vi "Helium Test - Step 2.vi"(7 "Step":i32, 8 "error in":errorcluster, 9 "Test Results":T9, 10 "Oil In":T1, 11 "Test Configuration":T2) -> (0 "error out":errorcluster, 1 "Test Results Out":T9, 2 "Oil Out":T1, 3 "Test Configuration Out":T2)   [LabVIEW 2015]
uses:
  Controls/Test Results.ctl
  Controls/Step Result.ctl
  Controls/Startup Test.ctl
  Controls/Test Information.ctl
  Controls/Vacuum Test.ctl
  Controls/Test Timing.ctl
  Controls/Vaccum Thresholds.ctl
  Controls/Helium Test.ctl
  Controls/Helium Thresholds.ctl
  Controls/Startup Thresholds.ctl
  CAN Communication/Oil/Typedefs/Session Handle.ctl
  CAN Communication/Oil/Oil.lvclass
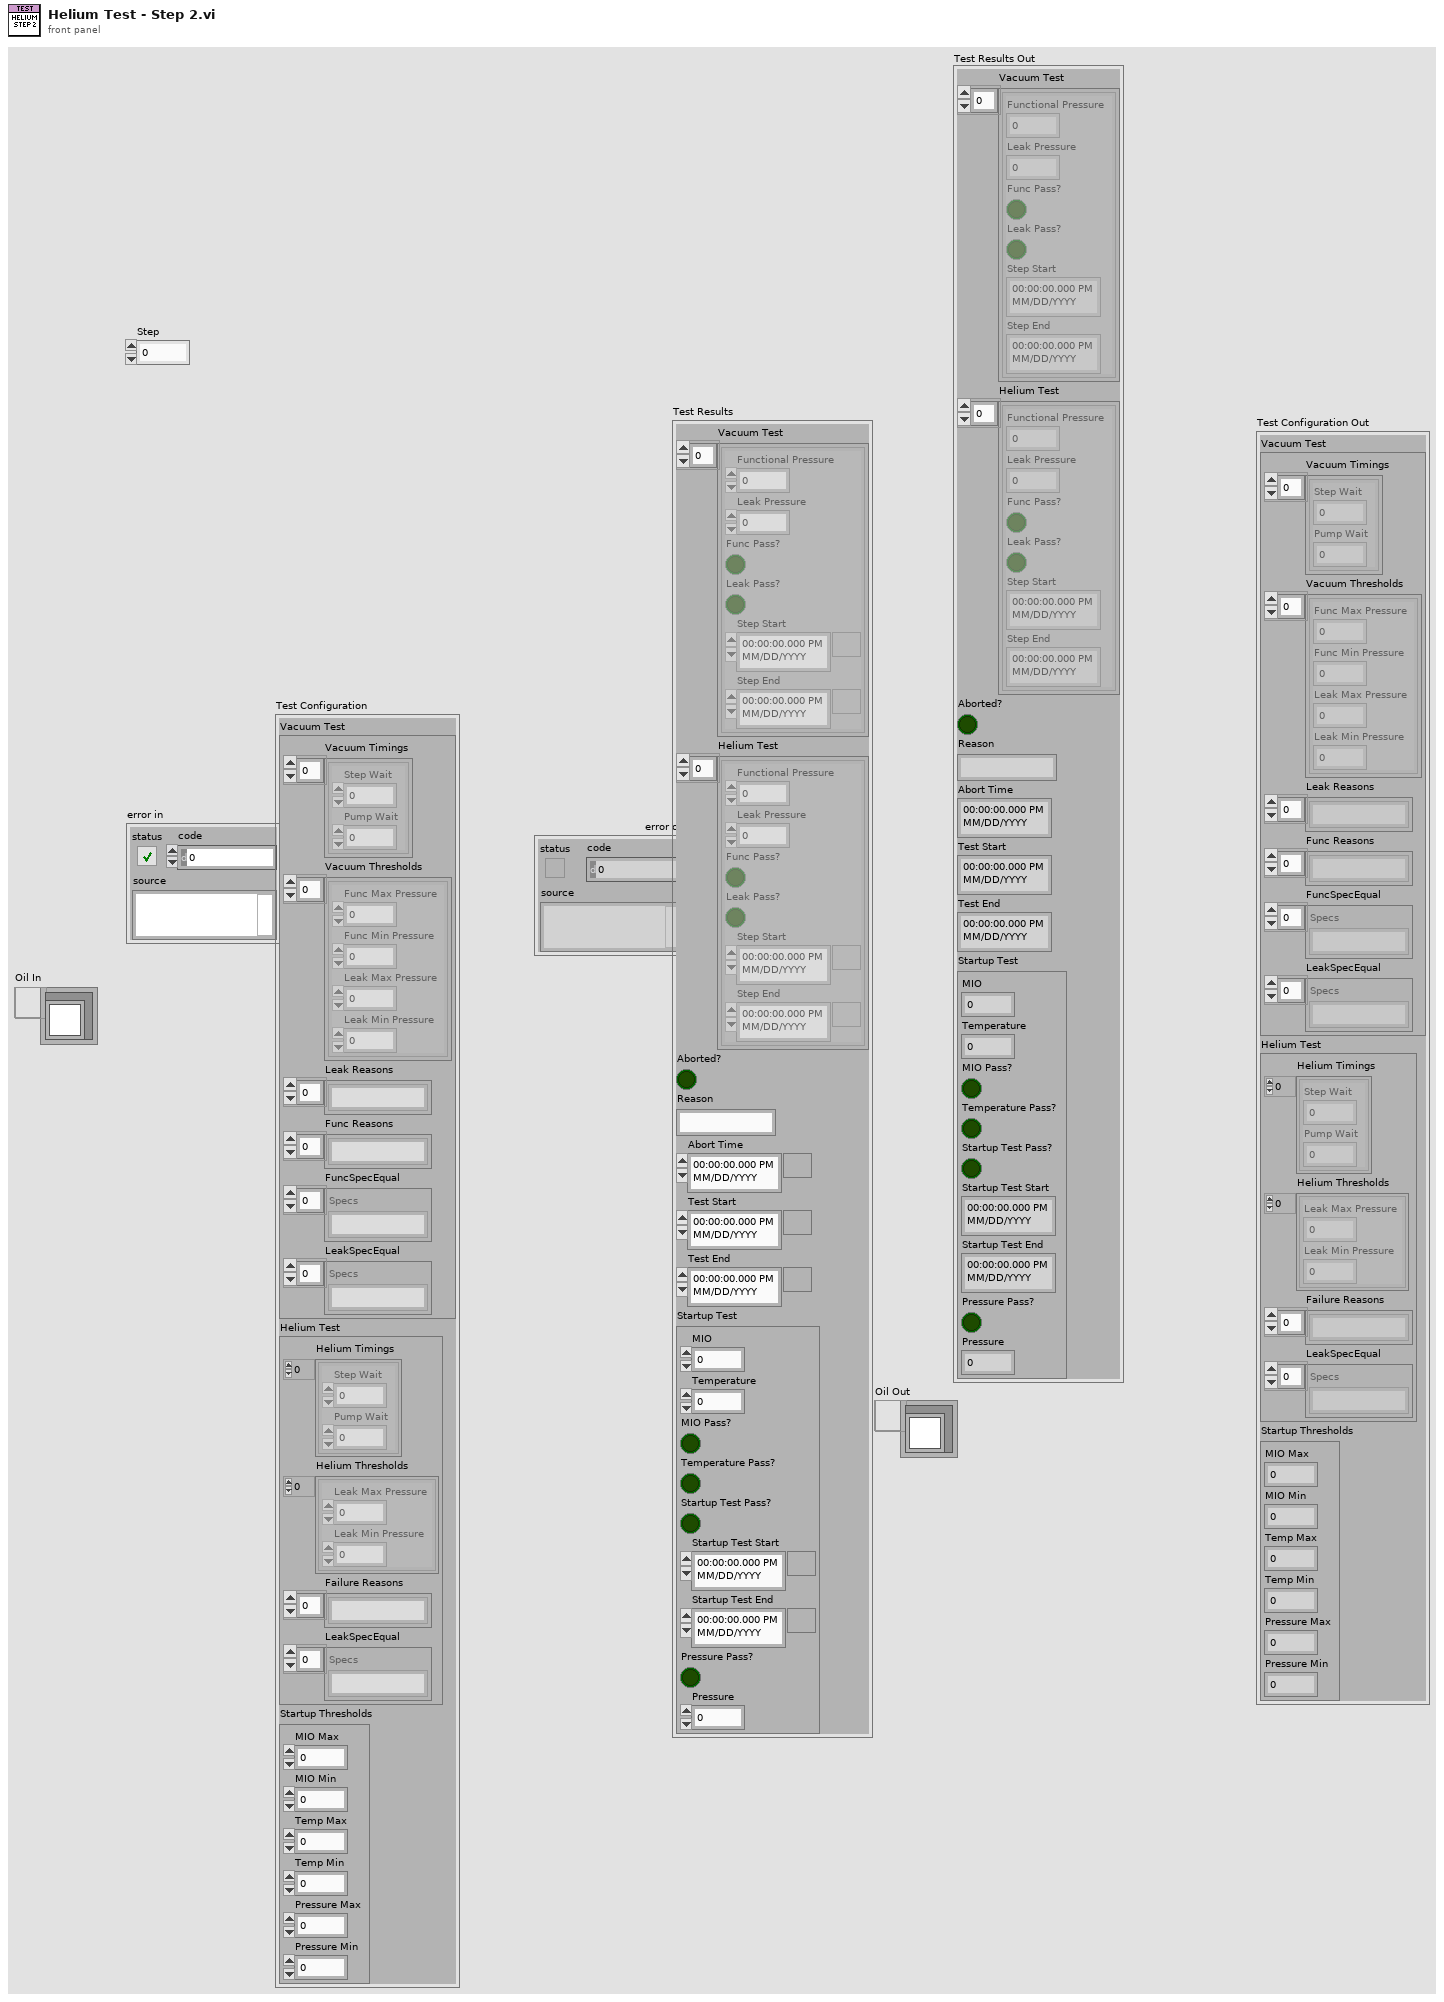
[diagram p1: front panel]
types:
  T1 = typedef "Oil.lvclass/Session Handle.ctl" = refnum<data-value>
  T2 = typedef "Test Information.ctl" = cluster{"Vacuum Test":T3, "Helium Test":T6, "Startup Thresholds":T8}
  T3 = typedef "Vacuum Test.ctl" = cluster{"Vacuum Timings":T4[], "Vacuum Thresholds":T5[], "Leak Reasons":string[], "Func Reasons":string[], "FuncSpecEqual":string[], "LeakSpecEqual":string[]}
  T4 = typedef "Test Timing.ctl" = cluster{"Step Wait":dbl, "Pump Wait":dbl}
  T5 = typedef "Vaccum Thresholds.ctl" = cluster{"Func Max Pressure":dbl, "Func Min Pressure":dbl, "Leak Max Pressure":dbl, "Leak Min Pressure":dbl}
  T6 = typedef "Helium Test.ctl" = cluster{"Helium Timings":T4[], "Helium Thresholds":T7[], "Failure Reasons":string[], "LeakSpecEqual":string[]}
  T7 = typedef "Helium Thresholds.ctl" = cluster{"Leak Max Pressure":dbl, "Leak Min Pressure":dbl}
  T8 = typedef "Startup Thresholds.ctl" = cluster{"MIO Max":dbl, "MIO Min":dbl, "Temp Max":dbl, "Temp Min":dbl, "Pressure Max":dbl, "Pressure Min":dbl}
  T9 = typedef "Test Results.ctl" = cluster{"Vacuum Test":T10[], "Helium Test":T10[], "Aborted?":bool, "Reason":string, "Abort Time":timestamp, "Test Start":timestamp, "Test End":timestamp, "Startup Test":T11}
  T10 = typedef "Step Result.ctl" = cluster{"Functional Pressure":dbl, "Leak Pressure":dbl, "Func Pass?":bool, "Leak Pass?":bool, "Step Start":timestamp, "Step End":timestamp}
  T11 = typedef "Startup Test.ctl" = cluster{"MIO":dbl, "Temperature":dbl, "MIO Pass?":bool, "Temperature Pass?":bool, "Startup Test Pass?":bool, "Startup Test Start":timestamp, "Startup Test End":timestamp, "Pressure Pass?":bool, "Pressure":dbl}
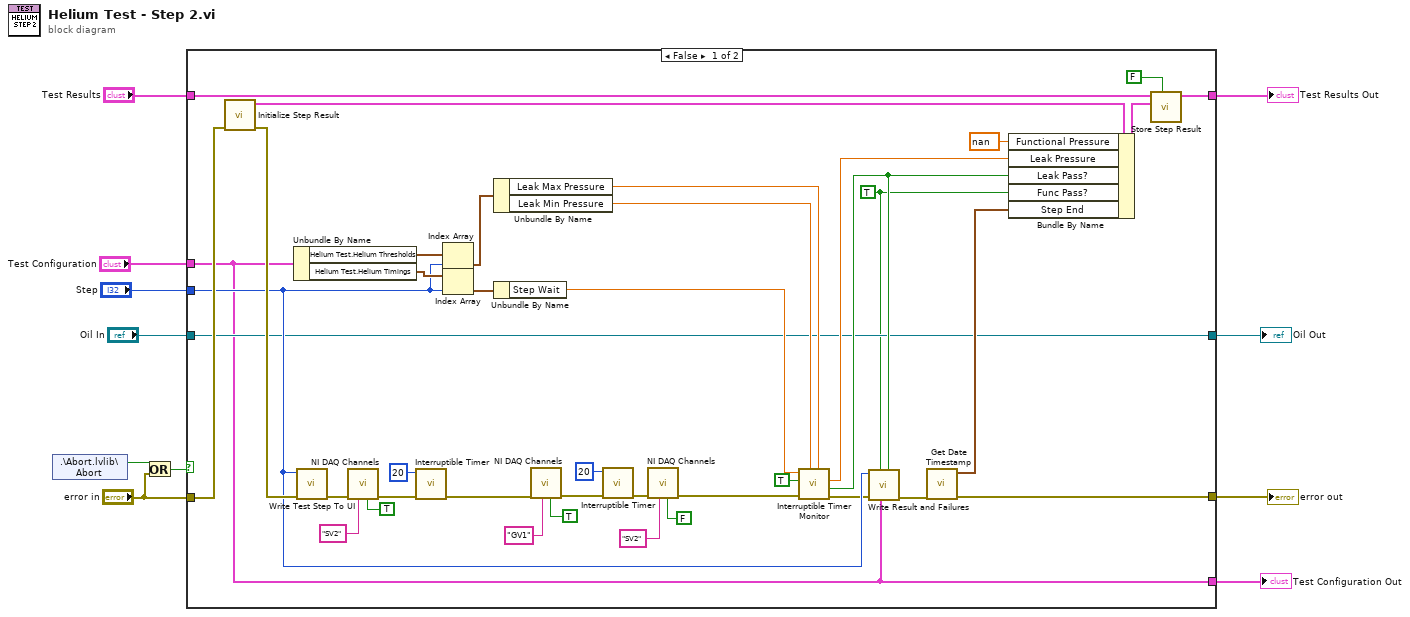
[diagram p0: block diagram]
diagram:
  n1 = shared-variable ".\\Abort.lvlib\\Abort"() -> (w10:bool)  [unwired: 1 in, 1 out]
  n2 = Or(x=w10, y="error in") -> (x .or. y?=w9:bool)
  n3 = case shown="False" w9 {
    tunnel: "error in" -> [w51 w54]
    tunnel: "Test Results" -> [w48 w55]
    tunnel: [w49 w55] -> w8
    tunnel: [w25 w54] -> w7
    tunnel: "Test Configuration" -> [w16 w53]
    tunnel: "Step" -> [w39 _]
    tunnel: [w16 w53] -> w3
    tunnel: [w26 w52] -> w1
    tunnel: "Oil In" -> [w26 w52]
    frame False {
      w23 = TRUE ("Func Pass?")
      n4 = call "Initialize Step Result.vi"("error in (no error)"=w51) -> ("error out"=w50:errorcluster, "New Step Result"=w47:T10)  [unwired: 8 in, 1 out]
      n5 = Unbundle By Name(w16) -> ("Helium Test.Helium Thresholds"=w44:T7[], "Helium Test.Helium Timings"=w43:T4[])
      n6 = call "Write Test Step To UI.vi"("error in (no error)"=w50, "Step"=w39) -> ("error out"=w37:errorcluster)  [unwired: 9 in]
      n7 = call "NI DAQ Channels.vi"("Control"=TRUE ("State"), "Channel"="SV2", "error in (no error)"=w37) -> ("error out"=w36:errorcluster)  [unwired: 7 in, 1 out]
      n8 = call "Interruptible Timer.vi"("error in (no error)"=w36, "Wait (s)"=20) -> ("error out"=w12:errorcluster)  [unwired: 7 in, 2 out]
      n9 = Index Array(array=w44, index=w39) -> (element=w40:T7)
      n10 = Index Array(array=w43, index=w39) -> (element=w42:T4)
      n11 = Unbundle By Name(w40) -> ("Leak Max Pressure"=w31:dbl, "Leak Min Pressure"=w32:dbl)
      n12 = Unbundle By Name(w42) -> ("Step Wait"=w34:dbl)
      n13 = call "NI DAQ Channels.vi"("Control"=TRUE ("State"), "Channel"="GV1", "error in (no error)"=w12) -> ("error out"=w21:errorcluster)  [unwired: 7 in, 1 out]
      n14 = call "Interruptible Timer.vi"("error in (no error)"=w21, "Wait (s)"=20) -> ("error out"=w19:errorcluster)  [unwired: 7 in, 2 out]
      n15 = call "NI DAQ Channels.vi"("Control"=FALSE ("State"), "Channel"="SV2", "error in (no error)"=w19) -> ("error out"=w17:errorcluster)  [unwired: 7 in, 1 out]
      n16 = call "Interruptible Timer Monitor.vi"("Max"=w31, "Min"=w32, "error in (no error)"=w17, "Update UI?"=TRUE, "Wait (s)"=w34) -> ("error out"=w28:errorcluster, "In Range?"=w29:bool, "Leak Rate"=w30:dbl)  [unwired: 2 in, 2 out]
      n17 = call "Write Result and Failures.vi"("Leak"=w29, "Test Configuration"=w16, "Func"=w23, "error in (no error)"=w28, "Step"=w39) -> ("error out"=w27:errorcluster)  [unwired: 6 in]
      n18 = call "Get Date Timestamp.vi"("error in (no error)"=w27) -> ("error out"=w25:errorcluster, "current time"=w45:timestamp)  [unwired: 9 in]
      n19 = Bundle By Name(cluster=w47, "Functional Pressure"=nan, "Leak Pressure"=w30, "Leak Pass?"=w29, "Func Pass?"=w23, "Step End"=w45) -> (w46:T10)
      n20 = call "Store Step Result.vi"("Vacuum?"=FALSE, "Step Result"=w46, "Test Results In"=w48) -> ("Test Results Out"=w49:T9)  [unwired: 8 in]
    }
    frame True {
    }
  }
  "error out" <- w7
  "Test Results Out" <- w8
  "Test Configuration Out" <- w3
  "Oil Out" <- w1
